vi "SaveAudioWaveformBlock.vi"(8 "error in (no error)":errorcluster, 10 "on demand waveform":T3, 11 "config":T2) -> (0 "error out":errorcluster, 1 "audio file complete":T1, 2 "complete":bool, 3 "config":T2)   [LabVIEW 2017, in "EmsaAudio.lvlib"]
uses:
  <vilib>/addons/InsightCM/Devices/Shared/Emsa/EmsaAudio/EmsaAudio.lvlib
  <vilib>/addons/InsightCM/Devices/Shared/Emsa/EmsaAcquisition/controls/OnDemandWaveformData.ctl
  <vilib>/addons/InsightCM/Devices/Shared/Emsa/EmsaAudio/controls/config.ctl
  <vilib>/addons/InsightCM/Devices/Shared/Emsa/EmsaAudio/controls/AudioFileCompleteBroadcast.ctl
  <vilib>/Waveform/WDTOps.llb/WDT Append Waveforms DBL.vi
  <vilib>/addons/InsightCM/Devices/Shared/Emsa/EmsaAcquisition/EmsaAcquisition.lvlib
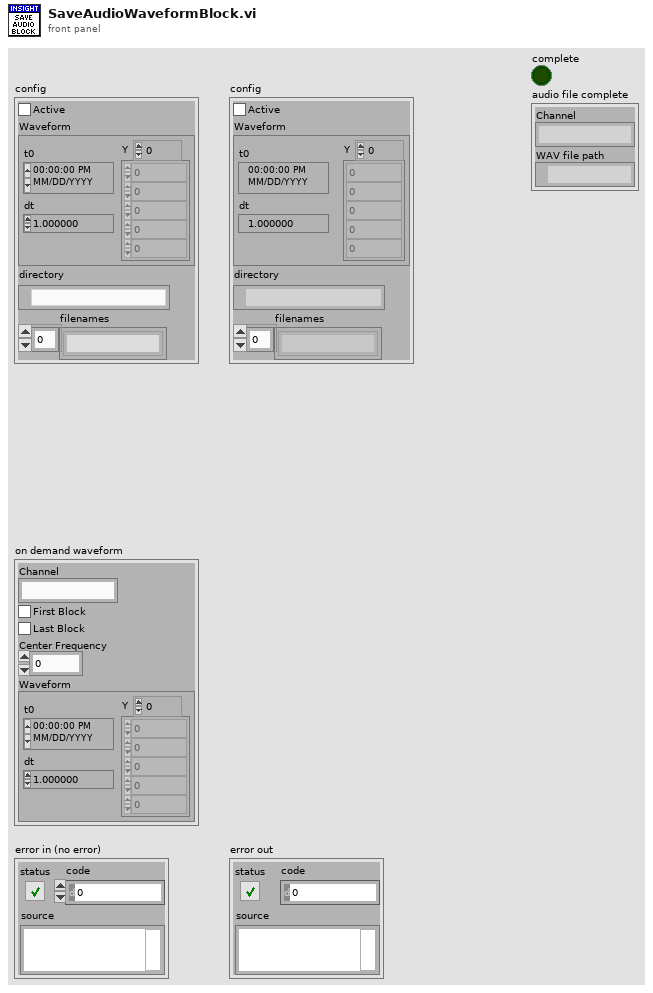
[diagram p1: front panel]
types:
  T1 = typedef "EmsaAudio.lvlib/AudioFileCompleteBroadcast.ctl" = cluster{"Channel":string, "WAV file path":path}
  T2 = typedef "EmsaAudio.lvlib/config.ctl" = cluster{"Active":bool, "Waveform":waveform(dbl), "directory":path, "filenames":string[]}
  T3 = typedef "EmsaAcquisition.lvlib/OnDemandWaveformData.ctl" = cluster{"Channel":string, "First Block":bool, "Last Block":bool, "Center Frequency":dbl, "Waveform":waveform(dbl)}
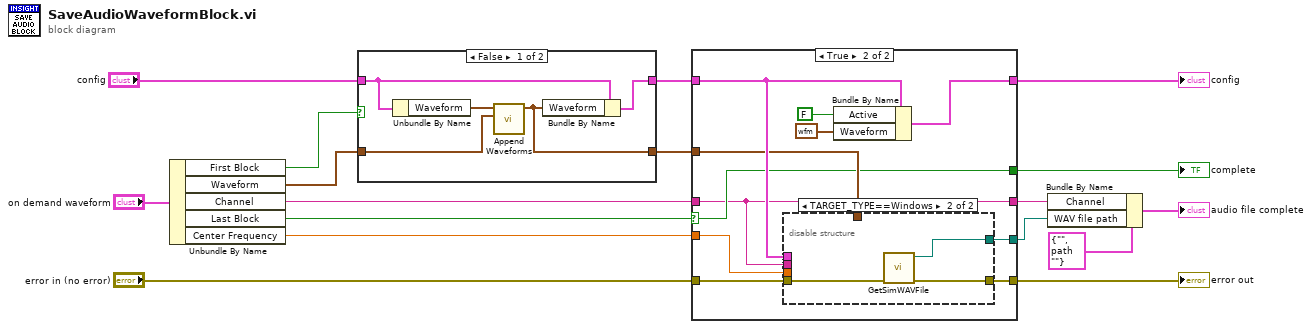
[diagram p0: block diagram]
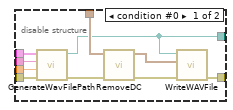
[diagram p3: hidden frame]
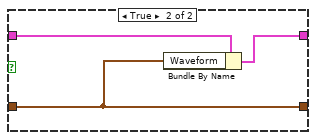
[diagram p4: hidden frame]
diagram:
  n1 = Unbundle By Name("on demand waveform") -> ("First Block"=w10:bool, "Waveform"=w12:waveform(dbl), "Channel"=w7:string, "Last Block"=w8:bool, "Center Frequency"=w15:dbl)
  n2 = case shown="False" w10 {
    tunnel: [w20 w24] -> w11
    tunnel: "config" -> [w21 w25]
    tunnel: w12 -> [w19 w23]
    tunnel: [w18 w23] -> w6
    frame False {
      n3 = Unbundle By Name(w21) -> ("Waveform"=w22:waveform(dbl))
      n4 = call-poly <vilib>:"Append Waveforms.vi"("waveform B"=w19, "waveform A"=w22) -> ("waveform out"=w18:waveform(dbl))  [unwired: 8 in, 1 out]
      n5 = Bundle By Name(cluster=w21, "Waveform"=w18) -> (w20:T2)
    }
    frame True {
      n6 = Bundle By Name(cluster=w25, "Waveform"=w23) -> (w24:T2)
    }
  }
  n7 = case shown="True" w8 {
    selector: w8 -> [w26 w31]
    tunnel: "error in (no error)" -> [w28 w39]
    tunnel: [w28 w38] -> w14
    tunnel: w15 -> [_ w37]
    tunnel: w11 -> [w27 w34]
    tunnel: [w27 w35] -> w16
    tunnel: w7 -> [_ w29]
    tunnel: w6 -> [_ w33]
    tunnel: [w26 w31] -> w5
    tunnel: [_ w30] -> w2
    tunnel: [_ w29] -> w3
    frame False {
    }
    frame True {
      n8 = disable-structure shown="TARGET_TYPE==Windows" {
        disable-tunnel: w39 -> [w49 w52]
        disable-tunnel: [w45 w51] -> w38
        disable-tunnel: w37 -> [w44 _]
        disable-tunnel: w34 -> [w43 _]
        disable-tunnel: w33 -> [w42 _]
        disable-tunnel: [w41 w50] -> w30
        disable-tunnel: w29 -> [w40 _]
        frame condition #0 {
          n9 = call <vilib>:"GenerateWavFilePath.vi"("error in (no error)"=w49, "center frequency"=w44, "Channel Name"=w40, "config"=w43) -> ("error out"=w48:errorcluster, "wav file path"=w41:path)  [unwired: 6 in]
          n10 = call <vilib>:"RemoveDC.vi"("error in (no error)"=w48, "waveform"=w42) -> ("error out"=w47:errorcluster, "waveform"=w46:waveform(dbl))  [unwired: 8 in]
          n11 = call <vilib>:"WriteWAVFile.vi"("error in (no error)"=w47, "Waveform"=w46, "Path"=w41) -> ("error out"=w45:errorcluster)  [unwired: 8 in]
        }
        frame condition #1 (active) {
          n12 = call <vilib>:"GetSimWAVFile.vi"("error in (no error)"=w52) -> ("error out"=w51:errorcluster, "wav file path"=w50:path)  [unwired: 9 in]
        }
      }
      n13 = Bundle By Name(cluster=w34, "Active"=FALSE, "Waveform"=waveform(dbl) {"t0"=timestamp(0 s since 1904-01-01), "dt"=1.0, "Y"=[]}) -> (w35:T2)
    }
  }
  "config" <- w16
  "error out" <- w14
  "complete" <- w5
  n14 = Bundle By Name(cluster=T1 {"Channel"="", "WAV file path"=path ""} ("Audio File Complete"), "Channel"=w3, "WAV file path"=w2) -> (→"audio file complete":T1)
